vi "SynthNV_2_5c.vi"() -> ()   [LabVIEW 2012]
uses:
  <vilib>/Utility/error.llb/DialogType.ctl
  <vilib>/Instr/_visa.llb/VISA Flush IO Buffer Mask.ctl
  <vilib>/Utility/file.llb/Read From Spreadsheet File (DBL).vi
  <vilib>/Instr/_visa.llb/VISA Configure Serial Port (Instr).vi
panel:
  out "Power (dBm)":dbl format="%#_4g"
  out "caldata":dbl[][](array[numeric]) format="%0.3f"
  out "COM Error":bool
  out "Device Under Control":string
  in  "Boolean":bool
  in  "Serial Port Select":refnum<visa-resource-name>="COM3"
  in  "Load":bool
  out "Lock":bool
  in  "RF HP":bool=TRUE
  in  "RF On":bool=TRUE
  in  "Dial Tab":enum32{"VFO Dial", "Touch Pad"}(tab)
  in  "Frequency Adjust":i8(knob)=1 scale=1.0..20.0
  in  "Knob Step Size":i32(ring)=3 items=["1KHz", "10KHz", "100KHz", "1MHz", "10MHz", "100MHz", "1GHz"]
  out "Freq (MHz) 3":dbl format="%#_7g"
  in  "KeyPad":T1
  out "KeyPad Out":dbl format="%7_7g"
  in  "Attenuator (dB)":dbl(slide)=-31.5 min=-31.5 max=0.0 step=0.5
  in  "stop":bool
  in  "Tab Control":T2(tab)
  in  "RF  FREQUENCY MHz":dbl=1000.0 min=34.375 max=4400.0 step=1.0 format="%_7g"
  in  "Enter":bool caption="1"
  out "PWR Level":bool
  out "Waveform Chart":dbl(graph)
  out "RF Detector Pwr dBm":dbl=-67.9609375 format="%_5g"
  in  "Read Power":bool
  in  "VREF":dbl=2.52 format="%#_7g"
  in  "POFFSET":dbl=97.0 format="%#_7g"
  in  "Send\nCal":bool
  in  "Start Network\nAnalyzer":bool
  out "Number\nof Points":dbl format="%#.6g"
  in  "Stop Frequency":dbl=4000.0 min=34.0 max=4400.0 step=0.001 format="%7_7g"
  in  "Step Time (mS)":dbl=0.55 min=0.25 max=10000.0 step=1.0 format="%_8g"
  in  "Step Size MHz":dbl=50.0 min=0.001 max=4200.0 step=1.0 format="%#_7f"
  in  "Enter SZ":bool caption="1"
  in  "Enter Start":bool caption="1"
  in  "Enter Stop":bool caption="1"
  in  "Enter ST":bool caption="1"
  in  "Start Frequency":dbl=50.0 min=34.0 max=4400.0 step=0.001 format="%7_7g"
  in  "Sweep\nOnce":bool
  in  "Sweep\nContinuously":bool
  in  "Mod Tab":enum32{"PULSE Amplitude", "AM"}(tab)
  in  "Mod Style":bool
  in  "PULNUM":bool caption="1"
  in  "PULOFF":bool caption="1"
  in  "PULON":bool caption="1"
  in  "Send Pulse Burst":bool
  out "Duration (uS)":dbl
  in  "Continuous PM":bool
  in  "# of Pulses":u16=100 min=1 step=1 format="%#.5f"
  in  "Off Time (uS)":u16=10 min=1 max=16000 step=1 format="%#.5f"
  in  "On Time (uS)":u16=1 min=1 max=16000 step=1 format="%#.5f"
  in  "AMAMP":bool caption="1"
  in  "AMPWR":bool caption="1"
  in  "AMCYC":bool caption="1"
  in  "AMFREQ":bool caption="1"
  in  "AM Freq (Hz)":dbl=1000.0 min=2.0 max=500000.0 step=10.0 format="%#.6f"
  out "Actual Freq (Hz)":dbl
  out "Duration (ms)":dbl
  in  "Send AM Burst":bool
  in  "# of Cycles":u16=100 min=1 step=1 format="%#.5f"
  in  "Offset":u8 max=62 step=1
  in  "Amplitude (%)":u8=100 min=1 max=100 step=1
  in  "Continuous AM":bool
  in  "Wave Shape":u8(ring) items=["Sine", "Ramp", "Triangle"]
  in  "LUTsize":u8=32 min=2 step=1
  in  "Read Settings\nFrom SynthNV":bool
  out "read buffer":string
  in  "Allow changing\nof Power Detector\ncalibration values":bool
  in  "GP Dig Out J8 P3":bool
  in  "Read A/D \non J8 P2":bool
  in  "Read A/D \non J8 P1":bool
  in  "REF":bool=TRUE
  in  "Program\nEEprom":bool
  in  "Read\nFirmware\nVersion":bool
  out "Version":string
  in  "Program\nReference":bool
  in  "Poll for\nPhase Lock":bool
  out "A/D1":string
  out "A/D2":string
  in  "GP Dig Out J8 P5":bool
  out "Frac":i32
  out "Modulus":i32=500
  out "INT":i16=2000
  out "RF Divider":i32=4
  out "Allregout":u32[](array[numeric])=[4194309, 10896444, 1203, 97986, 134254497, 65536000] format="%08x"
  out "PFd(MHz)":dbl=2.0
  in  "PllCntrl":T3={"PLL PWR"=3, "MUX out"=4, "Phase"=1, "Low Noise"=TRUE, "REF X2"=FALSE, "Mute till LD"=TRUE, "Icp"=15, "Band Sel Div"=16, "REF Divide"=5, "Reference(MHz)"=10.0} {"Icp" scale=0.0..15.0; "MUX out" items=["3-State", "GND", "Vcc", "Analog LD", "Digital LD", "REF / R", "RF / N"]; "PLL PWR" scale=0.0..3.0}
  in  "Step Size (MHz)":dbl=0.001
  in  "Send":bool
  in  "Freq (MHz)":dbl=1000.0 format="%_10g"
  in  "Re-init\nDefaults":bool
  # "v2.5c"
  # "Windfreak Technologies"
  # "MHz"
  # "Windfreak Technologies, LLC 2012"
  # "Warning: Max RF power into the\ndetector is 10dBm.  The Synthesizer\ncan generate up to +20dBm.  \nPlease use an external attenuator."
  # "Burst"
  # "Peak Amplitude is\nadjusted with slider\nbar on the right"
  # "Adjust Power Slider to get CW\npower back on after a pulse."
  # "Burst"
  # "(Or Update)"
  # "(Watch for LED D3 toggle.)"
  # "This Tab is for experimental purposes only."
  # "RF Freq (MHz)"
  # "REG5"
  # "REG4"
  # "REG3"
  # "REG2"
  # "REG1"
  # "REG0"
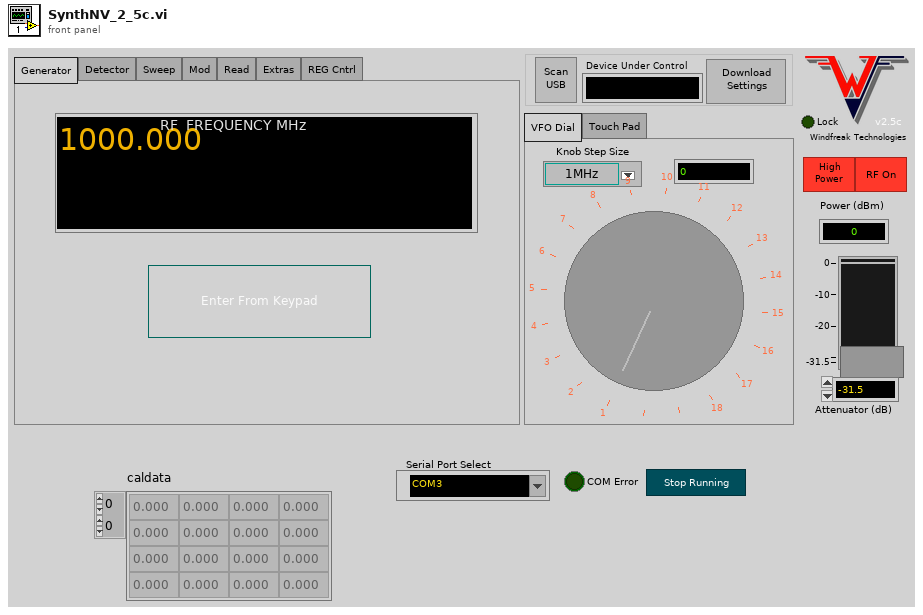
[diagram p1: front panel]
types:
  T1 = cluster{"2":bool, "1":bool, "3":bool, "4":bool, "9":bool, "5":bool, "6":bool, "7":bool, "8":bool, "0":bool, "dp":bool, "Clear":bool}
  T2 = enum32{"Generator", "Detector", "Sweep", "Mod", "Read", "Extras", "REG Cntrl"}
  T3 = cluster{"PLL PWR":i8, "MUX out":u16, "Phase":i16, "Low Noise":bool, "REF X2":bool, "Mute till LD":bool, "Icp":i32, "Band Sel Div":i32, "REF Divide":i16, "Reference(MHz)":dbl}
  T4 = enum8{"Enabled", "Disabled", "Disabled and Grayed Out"}
  T5 = typedef "DialogType.ctl" = u16
  T6 = typedef "VISA Flush IO Buffer Mask.ctl" = u16
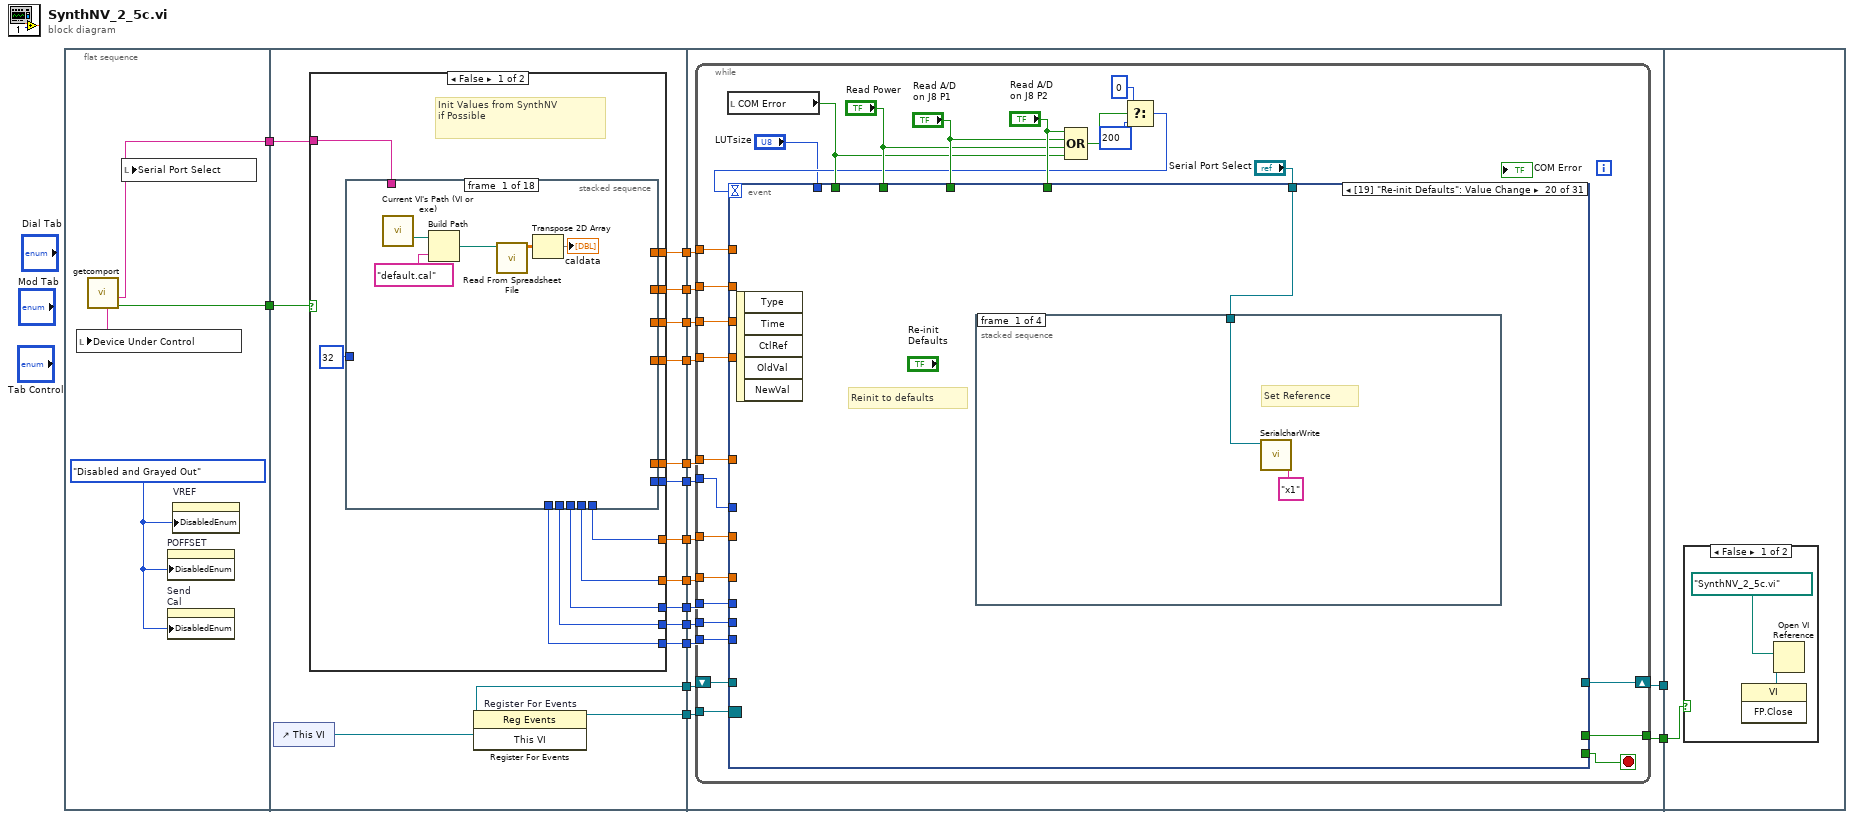
[diagram p0: block diagram]
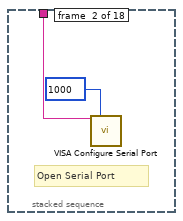
[diagram p2: hidden frame]
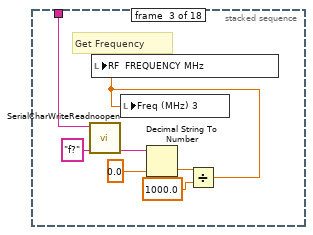
[diagram p3: hidden frame]
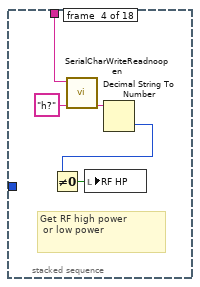
[diagram p4: hidden frame]
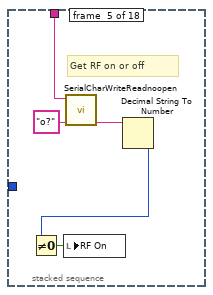
[diagram p5: hidden frame]
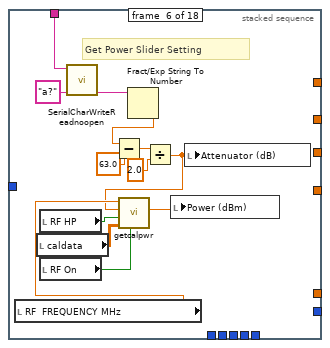
[diagram p6: hidden frame]
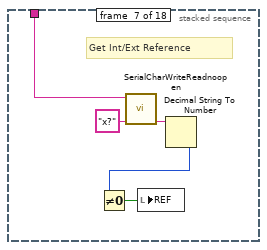
[diagram p7: hidden frame]
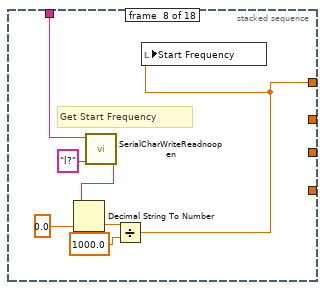
[diagram p8: hidden frame]
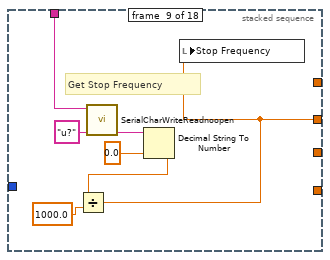
[diagram p9: hidden frame]
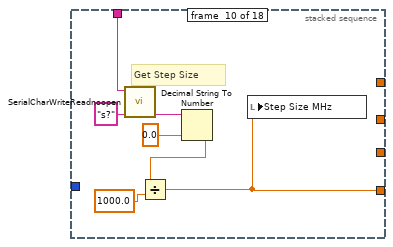
[diagram p10: hidden frame]
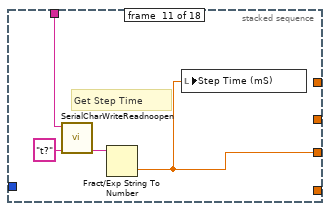
[diagram p11: hidden frame]
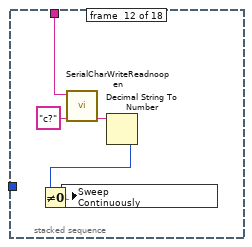
[diagram p12: hidden frame]
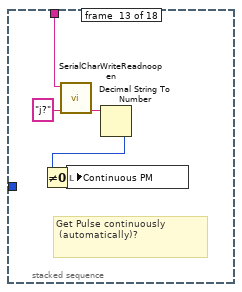
[diagram p13: hidden frame]
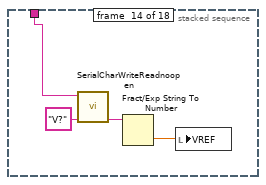
[diagram p14: hidden frame]
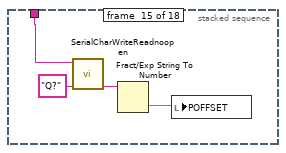
[diagram p15: hidden frame]
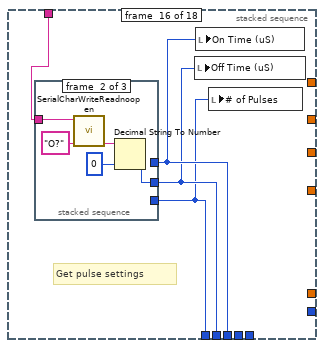
[diagram p16: hidden frame]
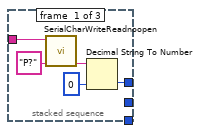
[diagram p17: hidden frame]
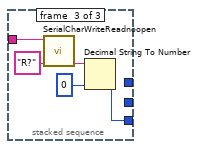
[diagram p18: hidden frame]
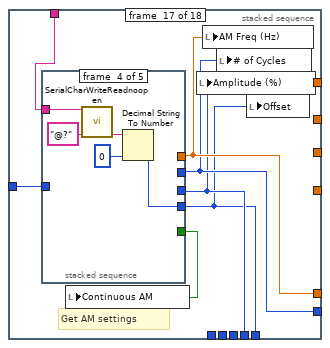
[diagram p19: hidden frame]
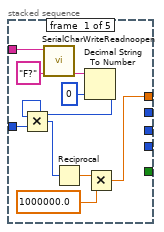
[diagram p20: hidden frame]
diagram:
  n1 = flat-sequence {
    tunnel: [w21] -> w17
    tunnel: [w20] -> w5
    tunnel: w17 -> [w36]
    tunnel: [w35] -> w16
    tunnel: [w34] -> w15
    tunnel: [w33] -> w14
    tunnel: [w32] -> w13
    tunnel: [w31] -> w12
    tunnel: [w30] -> w11
    tunnel: [w29] -> w10
    tunnel: [w28] -> w9
    tunnel: [w27] -> w8
    tunnel: [w26] -> w7
    tunnel: [w25] -> w6
    tunnel: w5 -> [w24]
    tunnel: [w22] -> w4
    tunnel: [w23] -> w3
    tunnel: w16 -> [w224]
    tunnel: w15 -> [w223]
    tunnel: w14 -> [w222]
    tunnel: w13 -> [w221]
    tunnel: w12 -> [w220]
    tunnel: w11 -> [w219]
    tunnel: w10 -> [w218]
    tunnel: w9 -> [w217]
    tunnel: w8 -> [w216]
    tunnel: w7 -> [w215]
    tunnel: w6 -> [w214]
    tunnel: w4 -> [w212]
    tunnel: w3 -> [w213]
    tunnel: [w211] -> w2
    tunnel: [w210] -> w1
    tunnel: w2 -> [_]
    tunnel: w1 -> [w887]
    frame #0 {
      w18 = T4."Disabled and Grayed Out" ("Disabled")
      n2 = call "getcomport.vi"() -> ("No Devices"=w21:bool, "Port"=w20:string, "Device"=w19:string)  [unwired: 9 in]
      n3 = local write "Device Under Control"(w19) -> ()
      n4 = local write "Serial Port Select"(w20) -> ()
      n5 = property on="POFFSET" class="DigNum (strict)"("DisabledEnum"=w18) -> ()  [unwired: 2 in, 2 out]
      n6 = property on="Send\nCal" class="Bool"("DisabledEnum"=w18) -> ()  [unwired: 2 in, 2 out]
      n7 = property on="VREF" class="DigNum (strict)"("DisabledEnum"=w18) -> ()  [unwired: 2 in, 2 out]
    }
    frame #1 {
      n8 = control-ref of="This VI"() -> (w23:refnum<vi>)
      n9 = case shown="False" w36 {
        tunnel: [w48 200.0 ("Start ini")] -> w35
        tunnel: [w47 4000.0 ("upper limit")] -> w34
        tunnel: [w45 u32 5 ("upper limit")] -> w33
        tunnel: [w46 50.0 ("upper limit")] -> w32
        tunnel: [w37 1000.0 ("Amp ini")] -> w31
        tunnel: [w38 u16 100 ("OnT ini")] -> w30
        tunnel: [w40 0.0 ("Amp ini")] -> w29
        tunnel: [w39 31.5 ("Amp ini")] -> w28
        tunnel: [w44 u16 1 ("OnT ini")] -> w27
        tunnel: [w42 u16 15 ("OnT ini")] -> w26
        tunnel: [w43 u16 100 ("OnT ini")] -> w25
        tunnel: w24 -> [w49 _]
        frame False {
          # "Init Values from SynthNV\nif Possible"
          n10 = stacked-sequence {
            tunnel: w49 -> [_ w56 w63 w65 w71 w84 w88 w93 w100 w107 w115 w118 w123 w128 w132 w138 w160 w192]
            tunnel: u8 32 ("LUTsize") -> [_ _ _ _ _ _ _ _ _ _ _ _ _ _ _ _ w159 _]
            tunnel: [_ _ _ _ _ _ _ w92 _ _ _ _ _ _ _ _ _ _] -> w48
            tunnel: [_ _ _ _ _ _ _ _ w99 _ _ _ _ _ _ _ _ _] -> w47
            tunnel: [_ _ _ _ _ _ _ _ _ w106 _ _ _ _ _ _ _ _] -> w46
            tunnel: [_ _ _ _ _ _ _ _ _ _ w113 _ _ _ _ _ _ _] -> w45
            tunnel: [_ _ _ _ _ _ _ _ _ _ _ _ _ _ _ w137 _ _] -> w44
            tunnel: [_ _ _ _ _ _ _ _ _ _ _ _ _ _ _ w135 _ _] -> w43
            tunnel: [_ _ _ _ _ _ _ _ _ _ _ _ _ _ _ w136 _ _] -> w42
            tunnel: [_ _ _ _ _ _ _ _ _ _ _ _ _ _ _ _ w154 _] -> w40
            tunnel: [_ _ _ _ _ _ _ _ _ _ _ _ _ _ _ _ w155 _] -> w39
            tunnel: [_ _ _ _ _ _ _ _ _ _ _ _ _ _ _ _ w156 _] -> w38
            tunnel: [_ _ _ _ _ _ _ _ _ _ _ _ _ _ _ _ w157 _] -> w37
            frame #0 {
              n11 = call "Current VI's Path (VI or exe).vi"() -> ("VI or executable installation directory"=w50:path)  [unwired: 14 in, 1 out]
              n12 = Build Path(base path=w50, name or relative path="default.cal") -> (appended path=w53:path)
              n13 = call-poly <vilib>:"Read From Spreadsheet File.vi"("file path (dialog if empty)"=w53) -> ("all rows"=w51:dbl[][])  [unwired: 6 in, 4 out]
              n14 = Transpose 2D Array(2D array=w51) -> (transposed array=→"caldata":dbl[][])
            }
            frame #1 {
              # "Open Serial Port"
              n15 = call-poly "VISA Configure Serial Port"("VISA resource name"=w56, "timeout (10sec)"=u32 1000) -> ()  [unwired: 7 in, 7 out]
            }
            frame #2 {
              # "Get Frequency"
              n16 = call "SerialCharWriteReadnoopen.vi"("VISA resource name"=w63, "write buffer"="f?") -> ("read buffer"=w61:string)  [unwired: 8 in]
              n17 = Decimal String To Number(string=w61, default (0L)=0.0 ("default (0 I32)")) -> (number=w59:dbl)  [unwired: 1 in, 1 out]
              n18 = Divide(x=w59, y=1000.0) -> (x/y=w57:dbl)
              n19 = local write "RF  FREQUENCY MHz"(w57) -> ()
              n20 = local write "Freq (MHz) 3"(w57) -> ()
            }
            frame #3 {
              # "Get RF high power\n or low power"
              n21 = call "SerialCharWriteReadnoopen.vi"("VISA resource name"=w65, "write buffer"="h?") -> ("read buffer"=w67:string)  [unwired: 8 in]
              n22 = Decimal String To Number(string=w67) -> (number=w66:i32)  [unwired: 2 in, 1 out]
              n23 = Not Equal To 0?(x=w66) -> (x != 0?=w64:bool)
              n24 = local write "RF HP"(w64) -> ()
            }
            frame #4 {
              # "Get RF on or off"
              n25 = call "SerialCharWriteReadnoopen.vi"("VISA resource name"=w71, "write buffer"="o?") -> ("read buffer"=w72:string)  [unwired: 8 in]
              n26 = Decimal String To Number(string=w72) -> (number=w70:i32)  [unwired: 2 in, 1 out]
              n27 = Not Equal To 0?(x=w70) -> (x != 0?=w69:bool)
              n28 = local write "RF On"(w69) -> ()
            }
            frame #5 {
              # "Get Power Slider Setting"
              n29 = local read "RF  FREQUENCY MHz"() -> (w78:dbl)
              n30 = local read "caldata"() -> (w79:dbl[][])
              n31 = local read "RF HP"() -> (w76:bool)
              n32 = local read "RF On"() -> (w75:bool)
              n33 = call "SerialCharWriteReadnoopen.vi"("VISA resource name"=w84, "write buffer"="a?") -> ("read buffer"=w85:string)  [unwired: 8 in]
              n34 = Fract/Exp String To Number(string=w85) -> (number=w80:dbl)  [unwired: 3 in, 1 out]
              n35 = Subtract(x=w80, y=63.0) -> (x-y=w81:dbl)
              n36 = Divide(x=w81, y=2.0) -> (x/y=w74:dbl)
              n37 = call "getcalpwr.vi"("RF On"=w75, "caldata"=w79, "RF HP"=w76, "attn"=w74, "freq"=w78) -> ("actual"=w77:dbl)  [unwired: 5 in]
              n38 = local write "Power (dBm)"(w77) -> ()
              n39 = local write "Attenuator (dB)"(w74) -> ()
            }
            frame #6 {
              # "Get Int/Ext Reference"
              n40 = call "SerialCharWriteReadnoopen.vi"("VISA resource name"=w88, "write buffer"="x?") -> ("read buffer"=w90:string)  [unwired: 8 in]
              n41 = Decimal String To Number(string=w90) -> (number=w89:i32)  [unwired: 2 in, 1 out]
              n42 = Not Equal To 0?(x=w89) -> (x != 0?=w87:bool)
              n43 = local write "REF"(w87) -> ()
            }
            frame #7 {
              # "Get Start Frequency"
              n44 = call "SerialCharWriteReadnoopen.vi"("VISA resource name"=w93, "write buffer"="l?") -> ("read buffer"=w97:string)  [unwired: 8 in]
              n45 = Decimal String To Number(string=w97, default (0L)=0.0 ("default (0 I32)")) -> (number=w95:dbl)  [unwired: 1 in, 1 out]
              n46 = Divide(x=w95, y=1000.0) -> (x/y=w92:dbl)
              n47 = local write "Start Frequency"(w92) -> ()
            }
            frame #8 {
              # "Get Stop Frequency"
              n48 = call "SerialCharWriteReadnoopen.vi"("VISA resource name"=w100, "write buffer"="u?") -> ("read buffer"=w104:string)  [unwired: 8 in]
              n49 = Decimal String To Number(string=w104, default (0L)=0.0 ("default (0 I32)")) -> (number=w102:dbl)  [unwired: 1 in, 1 out]
              n50 = Divide(x=w102, y=1000.0) -> (x/y=w99:dbl)
              n51 = local write "Stop Frequency"(w99) -> ()
            }
            frame #9 {
              # "Get Step Size"
              n52 = call "SerialCharWriteReadnoopen.vi"("VISA resource name"=w107, "write buffer"="s?") -> ("read buffer"=w111:string)  [unwired: 8 in]
              n53 = Decimal String To Number(string=w111, default (0L)=0.0 ("default (0 I32)")) -> (number=w109:dbl)  [unwired: 1 in, 1 out]
              n54 = Divide(x=w109, y=1000.0) -> (x/y=w106:dbl)
              n55 = local write "Step Size MHz"(w106) -> ()
            }
            frame #10 {
              # "Get Step Time"
              n56 = call "SerialCharWriteReadnoopen.vi"("VISA resource name"=w115, "write buffer"="t?") -> ("read buffer"=w114:string)  [unwired: 8 in]
              n57 = Fract/Exp String To Number(string=w114) -> (number=w113:dbl)  [unwired: 3 in, 1 out]
              n58 = local write "Step Time (mS)"(w113) -> ()
            }
            frame #11 {
              n59 = call "SerialCharWriteReadnoopen.vi"("VISA resource name"=w118, "write buffer"="c?") -> ("read buffer"=w120:string)  [unwired: 8 in]
              n60 = Decimal String To Number(string=w120) -> (number=w119:i32)  [unwired: 2 in, 1 out]
              n61 = Not Equal To 0?(x=w119) -> (x != 0?=w117:bool)
              n62 = local write "Sweep\nContinuously"(w117) -> ()
            }
            frame #12 {
              # "Get Pulse continuously\n (automatically)?"
              n63 = call "SerialCharWriteReadnoopen.vi"("VISA resource name"=w123, "write buffer"="j?") -> ("read buffer"=w125:string)  [unwired: 8 in]
              n64 = Decimal String To Number(string=w125) -> (number=w124:i32)  [unwired: 2 in, 1 out]
              n65 = Not Equal To 0?(x=w124) -> (x != 0?=w122:bool)
              n66 = local write "Continuous PM"(w122) -> ()
            }
            frame #13 {
              n67 = call "SerialCharWriteReadnoopen.vi"("VISA resource name"=w128, "write buffer"="V?") -> ("read buffer"=w129:string)  [unwired: 8 in]
              n68 = Fract/Exp String To Number(string=w129) -> (number=w127:dbl)  [unwired: 3 in, 1 out]
              n69 = local write "VREF"(w127) -> ()
            }
            frame #14 {
              n70 = call "SerialCharWriteReadnoopen.vi"("VISA resource name"=w132, "write buffer"="Q?") -> ("read buffer"=w133:string)  [unwired: 8 in]
              n71 = Fract/Exp String To Number(string=w133) -> (number=w131:dbl)  [unwired: 3 in, 1 out]
              n72 = local write "POFFSET"(w131) -> ()
            }
            frame #15 {
              # "Get pulse settings"
              n73 = stacked-sequence {
                tunnel: w138 -> [w141 w146 w151]
                tunnel: [w139 _ _] -> w137
                tunnel: [_ w145 _] -> w136
                tunnel: [_ _ w150] -> w135
                frame #0 {
                  n74 = call "SerialCharWriteReadnoopen.vi"("VISA resource name"=w141, "write buffer"="P?") -> ("read buffer"=w142:string)  [unwired: 8 in]
                  n75 = Decimal String To Number(string=w142, default (0L)=u16 0 ("default (0 I32)")) -> (number=w139:u16)  [unwired: 1 in, 1 out]
                }
                frame #1 {
                  n76 = call "SerialCharWriteReadnoopen.vi"("VISA resource name"=w146, "write buffer"="O?") -> ("read buffer"=w147:string)  [unwired: 8 in]
                  n77 = Decimal String To Number(string=w147, default (0L)=u16 0 ("default (0 I32)")) -> (number=w145:u16)  [unwired: 1 in, 1 out]
                }
                frame #2 {
                  n78 = call "SerialCharWriteReadnoopen.vi"("VISA resource name"=w151, "write buffer"="R?") -> ("read buffer"=w152:string)  [unwired: 8 in]
                  n79 = Decimal String To Number(string=w152, default (0L)=u16 0 ("default (0 I32)")) -> (number=w150:u16)  [unwired: 1 in, 1 out]
                }
              }
              n80 = local write "Off Time (uS)"(w136) -> ()
              n81 = local write "On Time (uS)"(w137) -> ()
              n82 = local write "# of Pulses"(w135) -> ()
            }
            frame #16 {
              # "Get AM settings"
              n83 = stacked-sequence {
                tunnel: w160 -> [w168 w173 w178 w182 w186]
                tunnel: [_ w172 _ _ _] -> w156
                tunnel: [_ _ w177 _ _] -> w155
                tunnel: [_ _ _ w181 _] -> w154
                tunnel: w159 -> [w166 _ _ _ _]
                tunnel: [w161 _ _ _ _] -> w157
                tunnel: [_ _ _ _ w187] -> w158
                frame #0 {
                  n84 = call "SerialCharWriteReadnoopen.vi"("VISA resource name"=w168, "write buffer"="F?") -> ("read buffer"=w169:string)  [unwired: 8 in]
                  n85 = Decimal String To Number(string=w169, default (0L)=u16 0 ("default (0 I32)")) -> (number=w165:u16)  [unwired: 1 in, 1 out]
                  n86 = Multiply(x=w165, y=w166) -> (x*y=w164:u16)
                  n87 = Reciprocal(x=w164) -> (1/x=w163:dbl)
                  n88 = Multiply(x=w163, y=1000000.0) -> (x*y=w161:dbl)
                }
                frame #1 {
                  n89 = call "SerialCharWriteReadnoopen.vi"("VISA resource name"=w173, "write buffer"="q?") -> ("read buffer"=w174:string)  [unwired: 8 in]
                  n90 = Decimal String To Number(string=w174, default (0L)=u16 0 ("default (0 I32)")) -> (number=w172:u16)  [unwired: 1 in, 1 out]
                }
                frame #2 {
                  n91 = call "SerialCharWriteReadnoopen.vi"("VISA resource name"=w178, "write buffer"="%?") -> ("read buffer"=w179:string)  [unwired: 8 in]
                  n92 = Decimal String To Number(string=w179, default (0L)=u16 0 ("default (0 I32)")) -> (number=w177:u16)  [unwired: 1 in, 1 out]
                }
                frame #3 {
                  n93 = call "SerialCharWriteReadnoopen.vi"("VISA resource name"=w182, "write buffer"="@?") -> ("read buffer"=w184:string)  [unwired: 8 in]
                  n94 = Decimal String To Number(string=w184, default (0L)=u16 0 ("default (0 I32)")) -> (number=w181:u16)  [unwired: 1 in, 1 out]
                }
                frame #4 {
                  # "Cont AM"
                  n95 = call "SerialCharWriteReadnoopen.vi"("VISA resource name"=w186, "write buffer"="A?") -> ("read buffer"=w189:string)  [unwired: 8 in]
                  n96 = Decimal String To Number(string=w189) -> (number=w190:i32)  [unwired: 2 in, 1 out]
                  n97 = Not Equal To 0?(x=w190) -> (x != 0?=w187:bool)
                }
              }
              n98 = local write "Continuous AM"(w158) -> ()
              n99 = local write "Amplitude (%)"(w155) -> ()
              n100 = local write "AM Freq (Hz)"(w157) -> ()
              n101 = local write "# of Cycles"(w156) -> ()
              n102 = local write "Offset"(w154) -> ()
            }
            frame #17 {
              w196 = T5 0 items=["no dialog", "OK message", "continue or stop message", "OK message + warnings", "continue/stop + warnings"] ("type of dialog (OK msg:1)")
              # "Close session to port."
              n103 = VISA Close(VISA resource name=w192) -> (error out=w197:errorcluster)  [unwired: 1 in]
              n104 = call <vilib>:"Simple Error Handler.vi"("type of dialog (OK msg:1)"=w196, "error in (no error)"=w197) -> ("error?"=w191:bool)  [unwired: 7 out]
              n105 = Equal?(x=w191, y=TRUE) -> (x = y?=w194:bool)
              n106 = case shown="True" w194 {
                tunnel: "Serial Port Error" ("message") -> [_ w198]
                frame False {
                }
                frame True {
                  n107 = Two Button Dialog(message=w198) -> ()  [unwired: 2 in, 1 out]
                }
              }
            }
          }
        }
        frame True {
        }
      }
      n108 = register-events "Register For Events"(w23) -> (reference out=w22:refnum<event-registration>)  [unwired: 2 in, 1 out]
    }
    frame #2 {
      n109 = while {
        tunnel: w223 -> [w250]
        tunnel: w222 -> [w249]
        tunnel: w221 -> [w248]
        tunnel: w224 -> [w247]
        tunnel: w220 -> [w246]
        tunnel: w219 -> [w245]
        tunnel: w218 -> [w240]
        tunnel: w217 -> [w244]
        tunnel: w216 -> [w243]
        tunnel: w215 -> [w242]
        tunnel: w214 -> [w241]
        shift-right: [w235] -> w211
        shift-left: w213 -> [w237]
        tunnel: w212 -> [w236]
        tunnel: [w234] -> w210
        stop <- w238 stop-if-true
        n110 = local read "COM Error"() -> (w228:bool)
        n111 = Compound Arithmetic op=OR("Read A/D \non J8 P2", "Read A/D \non J8 P1", "Read Power", w228) -> (w227:bool)
        n112 = Select(t=0, s=w227, f=200) -> (s? t:f=w226:i32)
        n113 = event shown="[19] \"Re-init Defaults\": Value Change" {
          selector: w236 -> [_ _ _ _ _ _ _ _ _ _ _ _ _ _ _ _ _ _ _ _ _ _ _ _ _ _ _ _ _ _ _]
          dyn-events: _ -> [_ _ _ _ _ _ _ _ _ _ _ _ _ _ _ _ _ _ _ _ _ _ _ _ _ _ _ _ _ _ _]
          timeout: w226 -> [_ _ _ _ _ _ _ _ _ _ _ _ _ _ _ _ _ _ _ _ _ _ _ _ _ _ _ _ _ _ _]
          tunnel: w250 -> [_ w300 _ _ _ _ _ _ _ _ _ _ _ _ _ _ _ _ _ _ _ _ _ _ _ _ _ _ _ _ _]
          tunnel: w249 -> [_ w299 _ _ _ _ _ _ _ _ _ _ _ _ _ _ _ _ _ _ _ _ _ _ _ _ _ _ _ _ _]
          tunnel: w248 -> [_ w298 _ _ _ _ _ _ _ _ _ _ _ _ _ _ _ _ _ _ _ _ _ _ _ _ _ _ _ _ _]
          tunnel: w247 -> [_ w297 _ _ _ _ _ _ _ _ _ _ _ _ _ _ _ _ _ _ _ _ _ _ _ _ _ _ _ _ _]
          tunnel: w246 -> [_ w276 _ _ _ _ _ _ _ _ _ _ _ _ _ _ _ _ _ _ _ _ _ _ _ _ _ _ _ _ _]
          tunnel: w245 -> [_ w275 _ _ _ _ _ _ _ _ _ _ _ _ _ _ _ _ _ _ _ _ _ _ _ _ _ _ _ _ _]
          tunnel: w244 -> [_ w274 _ _ _ _ _ _ _ _ _ _ _ _ _ _ _ _ _ _ _ _ _ _ _ _ _ _ _ _ _]
          tunnel: w243 -> [_ w267 _ _ _ _ _ _ _ _ _ _ _ _ _ _ _ _ _ _ _ _ _ _ _ _ _ _ _ _ _]
          tunnel: w242 -> [_ w268 _ _ _ _ _ _ _ _ _ _ _ _ _ _ _ _ _ _ _ _ _ _ _ _ _ _ _ _ _]
          tunnel: w241 -> [_ w273 _ _ _ _ _ _ _ _ _ _ _ _ _ _ _ _ _ _ _ _ _ _ _ _ _ _ _ _ _]
          tunnel: w240 -> [_ w270 _ _ _ _ _ _ _ _ _ _ _ _ _ _ _ _ _ _ _ _ _ _ _ _ _ _ _ _ _]
          tunnel: "Serial Port Select" -> [w263 _ w312 w327 w354 w401 w402 _ w415 w426 _ w437 w441 w449 w456 w462 w465 w474 w489 w565 w594 w595 w602 w605 w616 w625 w638 w650 _ _ w841]
          tunnel: [_ _ _ _ _ _ _ "stop" _ _ _ _ _ _ _ _ _ _ _ _ _ _ _ _ _ _ _ _ _ w835 _] -> w238
          tunnel: w237 -> [_ _ _ _ _ _ _ _ _ _ _ _ _ _ _ _ _ _ _ _ _ _ _ _ _ _ _ _ _ w834 _]
          tunnel: [_ _ _ _ _ _ _ _ _ _ _ _ _ _ _ _ _ _ _ _ _ _ _ _ _ _ _ _ _ w834 _] -> w235
          tunnel: [_ _ _ _ _ _ _ "stop" _ _ _ _ _ _ _ _ _ _ _ _ _ _ _ _ _ _ _ _ _ _ _] -> w234
          tunnel: w228 -> [_ _ _ _ _ _ _ _ _ _ _ _ _ _ _ _ _ _ _ _ _ _ _ _ _ _ _ _ _ _ w840]
          tunnel: "Read Power" -> [_ _ _ _ _ _ _ _ _ _ _ _ _ _ _ _ _ _ _ _ _ _ _ _ _ _ _ _ _ _ w839]
          tunnel: "Read A/D \non J8 P1" -> [_ _ _ _ _ _ _ _ _ _ _ _ _ _ _ _ _ _ _ _ _ _ _ _ _ _ _ _ _ _ w838]
          tunnel: "Read A/D \non J8 P2" -> [_ _ _ _ _ _ _ _ _ _ _ _ _ _ _ _ _ _ _ _ _ _ _ _ _ _ _ _ _ _ w837]
          tunnel: "LUTsize" -> [_ _ _ _ _ _ _ _ _ _ _ _ _ _ _ w457 w464 _ _ _ _ _ _ _ _ _ _ _ w670 _ _]
          event "Frequency Adjust", "RF  FREQUENCY MHz": Value Change {
            n114 = event-data() -> ()  [unwired: 1 in, 5 out]
            n115 = call "Knob.vi"("Freqin"="RF  FREQUENCY MHz", "Knob"="Frequency Adjust", "Knob Step Size"="Knob Step Size") -> ("Freqout"=w256:dbl)  [unwired: 7 in]
            "Freq (MHz) 3" <- w256
            n116 = local write "RF  FREQUENCY MHz"(w256) -> ()
            n117 = local read "Attenuator (dB)"() -> (w251:dbl)
            n118 = local read "caldata"() -> (w255:dbl[][])
            n119 = local read "RF HP"() -> (w253:bool)
            n120 = local read "RF On"() -> (w252:bool)
            n121 = Number To Fractional String(use system decimal point (T)=FALSE, number=w256, precision (6)=i16 3) -> (F-format string=w261:string)  [unwired: 1 in]
            n122 = call "getcalpwr.vi"("RF On"=w252, "caldata"=w255, "RF HP"=w253, "attn"=w251, "freq"=w256) -> ("actual"=w254:dbl)  [unwired: 5 in]
            n123 = Concatenate Strings("f" ("element"), w261) -> (w258:string)
            n124 = local write "Power (dBm)"(w254) -> ()
            n125 = call "SerialcharWrite.vi"("VISA resource name"=w263, "write buffer"=w258) -> ("ComError"=w262:bool)  [unwired: 8 in]
            n126 = local write "COM Error"(w262) -> ()
          }
          event "AMPWR", "AMCYC", "Enter Start", "Enter Stop", "Enter ST", "Enter SZ", "AMAMP", "AMFREQ", "PULNUM", "PULOFF", "PULON": Value Change {
            n127 = event-data() -> ()  [unwired: 1 in, 5 out]
            n128 = local read "KeyPad Out"() -> (w269:dbl)
            n129 = call "PulseModEntry.vi"("OnTimeSet"="PULON", "Keypad In"=w269, "OnT ini"=w267, "OffTimeSet"="PULOFF", "OffT ini"=w268, "PulsesSet"="PULNUM", "Pulses ini"=w273) -> ("OnTime"=w284:u16, "OffTime"=w283:u16, "NumPulses"=w271:u32)  [unwired: 4 in, 2 out]
            n130 = call "AMModEntry.vi"("AMFreqSet"="AMFREQ", "Keypad In"=w269, "AMFreq ini"=w276, "NumCycSet"="AMCYC", "NumCyc ini"=w275, "PkPwrSet"="AMPWR", "PkPwr ini"=w270, "AmpSet"="AMAMP", "Amp ini"=w274) -> ("AM Freq"=w288:dbl, "NumCyc"=w287:u16, "PkPwr"=w286:dbl, "Amplitude"=w285:dbl)  [unwired: 2 in, 1 out]
            n131 = call "SweepDataEntry.vi"("Enter Stop"="Enter Stop", "Start ini"=w297, "Enter Start"="Enter Start", "Keypad In"=w269, "Stop ini"=w300, "Enter ST"="Enter ST", "Step ini"=w299, "Enter SZ"="Enter SZ", "SZ ini"=w298) -> ("START FREQUENCY MHz"=w291:dbl, "STOP FREQUENCY MHz"=w292:dbl, "Step Time mS"=w293:dbl, "Step Size MHz"=w294:dbl)  [unwired: 2 in, 1 out]
            n132 = case shown="True" "Enter ST" {
              tunnel: w293 -> [_ w309]
              frame False {
              }
              frame True {
                n133 = local write "Step Time (mS)"(w309) -> ()
              }
            }
            n134 = case shown="True" "Enter SZ" {
              tunnel: w294 -> [_ w308]
              frame False {
              }
              frame True {
                n135 = local write "Step Size MHz"(w308) -> ()
              }
            }
            n136 = case shown="True" "Enter Start" {
              tunnel: w291 -> [_ w311]
              frame False {
              }
              frame True {
                n137 = local write "Start Frequency"(w311) -> ()
              }
            }
            n138 = case shown="True" "Enter Stop" {
              tunnel: w292 -> [_ w310]
              frame False {
              }
              frame True {
                n139 = local write "Stop Frequency"(w310) -> ()
              }
            }
            n140 = case shown="True" "AMAMP" {
              tunnel: w285 -> [_ w304]
              frame False {
              }
              frame True {
                n141 = local write "Amplitude (%)"(w304) -> ()
              }
            }
            n142 = case shown="True" "AMFREQ" {
              tunnel: w288 -> [_ w307]
              frame False {
              }
              frame True {
                n143 = local write "AM Freq (Hz)"(w307) -> ()
              }
            }
            n144 = case shown="True" "AMCYC" {
              tunnel: w287 -> [_ w306]
              frame False {
              }
              frame True {
                n145 = local write "# of Cycles"(w306) -> ()
              }
            }
            n146 = case shown="True" "AMPWR" {
              tunnel: w286 -> [_ w305]
              frame False {
              }
              frame True {
                n147 = local write "Offset"(w305) -> ()
              }
            }
            n148 = case shown="True" "PULON" {
              tunnel: w284 -> [_ w303]
              frame False {
              }
              frame True {
                n149 = local write "On Time (uS)"(w303) -> ()
              }
            }
            n150 = case shown="True" "PULOFF" {
              tunnel: w283 -> [_ w302]
              frame False {
              }
              frame True {
                n151 = local write "Off Time (uS)"(w302) -> ()
              }
            }
            n152 = case shown="True" "PULNUM" {
              tunnel: w271 -> [_ w301]
              frame False {
              }
              frame True {
                n153 = local write "# of Pulses"(w301) -> ()
              }
            }
          }
          event "KeyPad", "Enter": Value Change {
            n154 = event-data() -> ()  [unwired: 1 in, 5 out]
            n155 = call "Keypad.vi"("KeyPad"="KeyPad") -> ("Keypad Out"=w313:dbl)  [unwired: 14 in]
            "KeyPad Out" <- w313
            n156 = case shown="True" "Enter" {
              tunnel: w313 -> [_ w326]
              tunnel: w312 -> [_ w318]
              frame False {
              }
              frame True {
                n157 = In Range and Coerce(upper limit=4500.0, x=w326, lower limit=34.0) -> (coerced(x)=w316:dbl)  [unwired: 1 out]
                n158 = local write "RF  FREQUENCY MHz"(w316) -> ()
                n159 = local write "Freq (MHz) 3"(w316) -> ()
                n160 = Number To Fractional String(use system decimal point (T)=FALSE, number=w316, precision (6)=i16 3) -> (F-format string=w323:string)  [unwired: 1 in]
                n161 = Concatenate Strings("f" ("element"), w323) -> (w320:string)
                n162 = call "SerialcharWrite.vi"("VISA resource name"=w318, "write buffer"=w320) -> ("ComError"=w317:bool)  [unwired: 8 in]
                n163 = local write "COM Error"(w317) -> ()
              }
            }
          }
          event "Start Frequency", "Stop Frequency", "Step Time (mS)", "Step Size MHz": Value Change {
            # "Set up processor controlled Sweep\nand computer controlled sweep parameters"
            n164 = event-data() -> ()  [unwired: 1 in, 5 out]
            n165 = Subtract(x="Stop Frequency", y="Start Frequency") -> (x-y=w331:dbl)
            n166 = Divide(x=w331, y="Step Size MHz") -> (x/y=→"Number\nof Points":dbl)
            n167 = Number To Fractional String(use system decimal point (T)=FALSE, number="Step Size MHz", precision (6)=i16 3) -> (F-format string=w339:string)  [unwired: 1 in]
            n168 = Number To Fractional String(use system decimal point (T)=FALSE, number="Step Time (mS)", precision (6)=i16 3) -> (F-format string=w335:string)  [unwired: 1 in]
            n169 = Number To Fractional String(use system decimal point (T)=FALSE, number="Start Frequency", precision (6)=i16 3) -> (F-format string=w352:string)  [unwired: 1 in]
            n170 = Number To Fractional String(use system decimal point (T)=FALSE, number="Stop Frequency", precision (6)=i16 3) -> (F-format string=w343:string)  [unwired: 1 in]
            n171 = Concatenate Strings("d0" ("element"), "r0" ("string"), "l" ("element"), w352, "u" ("element"), w343, "s" ("element"), w339, "t" ("element"), w335) -> (w349:string)
            n172 = call "SerialcharWrite.vi"("VISA resource name"=w327, "write buffer"=w349) -> ("ComError"=w353:bool)  [unwired: 8 in]
            n173 = local write "COM Error"(w353) -> ()
          }
          event "On Time (uS)", "Off Time (uS)", "# of Pulses", "Mod Style": Value Change {
            w376 = 500000.0 ("y")
            # "Pulse Modulation"
            n174 = event-data() -> ()  [unwired: 1 in, 5 out]
            n175 = case shown="False" "Mod Style" {
              tunnel: [w380 u8 64] -> w378
              frame False {
                # "(only PDBrf is toggled)"
                # "High Symetry"
                n176 = local read "Attenuator (dB)"() -> (w381:dbl)
                n177 = Multiply(x=w381, y=2.0) -> (x*y=w383:dbl)
                n178 = Add(x=w383, y=63.0) -> (x+y=w385:dbl)
                n179 = To Unsigned Byte Integer(number=w385) -> (unsigned 8bit integer=w380:u8)
              }
              frame True {
                # "PDBrf plus DVGA lines\nare all toggled"
                # "Hi Isolation\nPAM"
              }
            }
            n180 = To Double Precision Float(number="On Time (uS)") -> (double precision float=w362:dbl)
            n181 = To Double Precision Float(number="Off Time (uS)") -> (double precision float=w361:dbl)
            n182 = To Double Precision Float(number="# of Pulses") -> (double precision float=w360:dbl)
            n183 = Add(x=w362, y=w361) -> (x+y=w375:dbl)
            n184 = Number To Decimal String(number="On Time (uS)") -> (decimal integer string=w357:string)  [unwired: 1 in]
            n185 = Number To Decimal String(number="Off Time (uS)") -> (decimal integer string=w358:string)  [unwired: 1 in]
            n186 = Number To Decimal String(number=w378) -> (decimal integer string=w365:string)  [unwired: 1 in]
            n187 = Multiply(x=w375, y=w360) -> (x*y=w371:dbl)
            n188 = Greater?(x=w371, y=w376) -> (0:w373:bool)
            n189 = case shown="True" w373 {
              tunnel: [w387 w389] -> w372
              tunnel: "# of Pulses" -> [w387 _]
              tunnel: w375 -> [_ w390]
              frame False {
              }
              frame True {
                n190 = Divide(x=500000.0 ("y"), y=w390) -> (x/y=w388:dbl)
                n191 = To Unsigned Word Integer(number=w388) -> (unsigned 16bit integer=w389:u16)
              }
            }
            n192 = Number To Decimal String(number=w372) -> (decimal integer string=w359:string)  [unwired: 1 in]
            n193 = Concatenate Strings("P" ("string"), w357, "O" ("string"), w358, "R" ("string"), w359, "M" ("string"), w365) -> (w366:string)
            n194 = call "SerialcharWrite.vi"("VISA resource name"=w354, "write buffer"=w366) -> ("ComError"=w379:bool)  [unwired: 8 in]
            n195 = local write "COM Error"(w379) -> ()
            n196 = In Range and Coerce(upper limit=w376, x=w371, lower limit=0.0) -> (coerced(x)=→"Duration (uS)":dbl)  [unwired: 1 out]
          }
          event "Sweep\nContinuously": Value Change {
            # "Sweep Continuously"
            n197 = event-data() -> ()  [unwired: 1 in, 5 out]
            n198 = Boolean To (0,1)(Boolean="Sweep\nContinuously") -> (0, 1=w400:i16)
            n199 = Number To Decimal String(number=w400) -> (decimal integer string=w396:string)  [unwired: 1 in]
            n200 = Concatenate Strings("d" ("element"), "0" ("element"), "c" ("element"), w396, "g" ("element"), w396) -> (w397:string)
            n201 = call "SerialcharWrite.vi"("VISA resource name"=w401, "write buffer"=w397) -> ("ComError"=w393:bool)  [unwired: 8 in]
            n202 = local write "COM Error"(w393) -> ()
          }
          event "Send\nCal": Value Change {
            n203 = event-data() -> ()  [unwired: 1 in, 5 out]
            n204 = Number To Fractional String(use system decimal point (T)=FALSE, number="VREF", precision (6)=i16 3) -> (F-format string=w409:string)  [unwired: 1 in]
            n205 = Number To Fractional String(use system decimal point (T)=FALSE, number="POFFSET", precision (6)=i16 3) -> (F-format string=w404:string)  [unwired: 1 in]
            n206 = Concatenate Strings("V" ("element"), w409, "Q" ("string"), w404) -> (w412:string)
            n207 = call "SerialcharWrite.vi"("VISA resource name"=w402, "write buffer"=w412) -> ()  [unwired: 8 in, 1 out]
          }
          event "stop": Value Change {
            n208 = event-data() -> ()  [unwired: 1 in, 5 out]
          }
          event "Read Settings\nFrom SynthNV": Value Change {
            n209 = event-data() -> ()  [unwired: 1 in, 5 out]
            n210 = call "SerialCharWriteandRead.vi"("VISA resource name"=w415, "write buffer"="?") -> ("error?"=w416:bool, "read buffer"=→"read buffer":string)  [unwired: 5 in, 2 out]
            n211 = local write "COM Error"(w416) -> ()
          }
          event "Sweep\nOnce": Value Change {
            # "Sweep Once"
            n212 = event-data() -> ()  [unwired: 1 in, 5 out]
            n213 = local read "Stop Frequency"() -> (w419:dbl)
            n214 = Concatenate Strings("d" ("element"), "0" ("element"), "g" ("element"), "1" ("string")) -> (w423:string)
            n215 = call "SerialcharWrite.vi"("VISA resource name"=w426, "write buffer"=w423) -> ("ComError"=w420:bool)  [unwired: 8 in]
            n216 = local write "COM Error"(w420) -> ()
            n217 = local write "RF  FREQUENCY MHz"(w419) -> ()
            n218 = local write "Freq (MHz) 3"(w419) -> ()
          }
          event "Allow changing\nof Power Detector\ncalibration values": Value Change {
            n219 = event-data() -> ()  [unwired: 1 in, 5 out]
            n220 = Select(t=T4."Enabled" ("Disabled"), s="Allow changing\nof Power Detector\ncalibration values", f=T4."Disabled and Grayed Out" ("Disabled")) -> (s? t:f=w428:T4)
            n221 = property on="Send\nCal" class="Bool"("DisabledEnum"=w428) -> ()  [unwired: 2 in, 2 out]
            n222 = property on="VREF" class="DigNum (strict)"("DisabledEnum"=w428) -> ()  [unwired: 2 in, 2 out]
            n223 = property on="POFFSET" class="DigNum (strict)"("DisabledEnum"=w428) -> ()  [unwired: 2 in, 2 out]
          }
          event "Continuous PM": Value Change {
            # "Pulse Continuously"
            n224 = event-data() -> ()  [unwired: 1 in, 5 out]
            n225 = Boolean To (0,1)(Boolean="Continuous PM") -> (0, 1=w436:i16)
            n226 = Select(t=2.0, s="Continuous PM", f=0.0) -> (s? t:f=w440:dbl)
            n227 = property on="Send Pulse Burst" class="Bool"("DisabledEnum"=w440) -> ()  [unwired: 2 in, 2 out]
            n228 = Number To Decimal String(number=w436) -> (decimal integer string=w433:string)  [unwired: 1 in]
            n229 = Concatenate Strings("j" ("element"), w433) -> (w434:string)
            n230 = call "SerialcharWrite.vi"("VISA resource name"=w437, "write buffer"=w434) -> ("ComError"=w432:bool)  [unwired: 8 in]
            n231 = local write "COM Error"(w432) -> ()
          }
          event "Send Pulse Burst": Value Change {
            # "Send Pulse Burst"
            n232 = event-data() -> ()  [unwired: 1 in, 5 out]
            n233 = call "SerialcharWrite.vi"("VISA resource name"=w441, "write buffer"="G") -> ("ComError"=w443:bool)  [unwired: 8 in]
            n234 = local write "COM Error"(w443) -> ()
          }
          event "Continuous AM": Value Change {
            n235 = event-data() -> ()  [unwired: 1 in, 5 out]
            n236 = Select(t=2.0, s="Continuous AM", f=0.0) -> (s? t:f=w452:dbl)
            n237 = property on="Send AM Burst" class="Bool"("DisabledEnum"=w452) -> ()  [unwired: 2 in, 2 out]
            n238 = Boolean To (0,1)(Boolean="Continuous AM") -> (0, 1=w448:i16)
            n239 = Number To Decimal String(number=w448) -> (decimal integer string=w445:string)  [unwired: 1 in]
            n240 = Concatenate Strings("A" ("element"), w445) -> (w446:string)
            n241 = call "SerialcharWrite.vi"("VISA resource name"=w449, "write buffer"=w446) -> ("ComError"=w444:bool)  [unwired: 8 in]
            n242 = local write "COM Error"(w444) -> ()
          }
          event "Send AM Burst": Value Change {
            n243 = event-data() -> ()  [unwired: 1 in, 5 out]
            n244 = call "SerialcharWrite.vi"("VISA resource name"=w456, "write buffer"="B") -> ("ComError"=w454:bool)  [unwired: 8 in]
            n245 = local write "COM Error"(w454) -> ()
          }
          event "LUTsize", "Wave Shape": Value Change {
            # "AM"
            # "Setup Lookup Table for AM"
            n246 = event-data() -> ()  [unwired: 1 in, 5 out]
            n247 = call "AMLUTwaveselect.vi"("Wave Shape"="Wave Shape", "LUTsize"=w457) -> ("Array"=w459:u8[])  [unwired: 1 in]
            n248 = Build Array (concatenate)(u8 9 ("element"), w457, w459) -> (w461:u8[])
            n249 = call "SerialByteWrite.vi"("VISA resource name"=w462, "unsigned byte array"=w461) -> ("error?"=w458:bool)  [unwired: 8 in]
            n250 = local write "COM Error"(w458) -> ()
          }
          event "AM Freq (Hz)", "# of Cycles", "Amplitude (%)", "Offset": Value Change {
            n251 = event-data() -> ()  [unwired: 1 in, 5 out]
            n252 = call "AMFreqminduration.vi"("Offset"="Offset", "Amplitude (%)"="Amplitude (%)", "Reps"="# of Cycles", "AM Freq (Hz)"="AM Freq (Hz)", "LUT size"=w464) -> ("Duration (ms)"=→"Duration (ms)":dbl, "AMout"=w473:string, "Actual Freq"=→"Actual Freq (Hz)":dbl)  [unwired: 4 in]
            n253 = call "SerialcharWrite.vi"("VISA resource name"=w465, "write buffer"=w473) -> ("ComError"=w466:bool)  [unwired: 8 in]
            n254 = local write "COM Error"(w466) -> ()
          }
          event "PllCntrl", "Send", "Freq (MHz)", "Step Size (MHz)": Value Change {
            # "RAW register writes for controlling\nregisters 2,3,5 especially"
            n255 = event-data() -> ()  [unwired: 1 in, 5 out]
            n256 = call "Getsettings.vi"("PllCntrl"="PllCntrl", "Step Size  (MHz)"="Step Size (MHz)", "Freq (MHz)"="Freq (MHz)") -> ("Modulus"=w479:i32, "INT"=w478:i16, "FRAC"=w477:i32, "RF Divider"=w476:i32, "Pfd (MHz)"=→"PFd(MHz)":dbl)  [unwired: 1 in, 2 out]
            "Frac" <- w477
            "Modulus" <- w479
            "INT" <- w478
            "RF Divider" <- w476
            n257 = call "Get Registers.vi"("Out Divider"=w476, "PllCntrl"="PllCntrl", "INT"=w478, "FRAC"=w477, "MOD"=w479) -> ("concatenated string"=w482:string, "Allregout"=→"Allregout":u32[])  [unwired: 13 in]
            n258 = case shown="True" "Send" {
              tunnel: w474 -> [_ w488]
              tunnel: w482 -> [_ w487]
              frame False {
              }
              frame True {
                n259 = call "SerialcharWrite.vi"("VISA resource name"=w488, "write buffer"=w487) -> ("ComError"=w486:bool)  [unwired: 8 in]
                n260 = local write "COM Error"(w486) -> ()
              }
            }
          }
          event "Start Network\nAnalyzer": Value Change {
            n261 = event-data() -> ()  [unwired: 1 in, 5 out]
            n262 = stacked-sequence {
              tunnel: w489 -> [w491 _ _ _ w519 w532 w534]
              frame #0 {
                n263 = local read "Attenuator (dB)"() -> (w492:dbl)
                n264 = Multiply(x=w492, y=2.0) -> (x*y=w498:dbl)
                n265 = Add(x=w498, y=63.0) -> (x+y=w500:dbl)
                n266 = To Unsigned Byte Integer(number=w500) -> (unsigned 8bit integer=w493:u8)
                n267 = Number To Decimal String(number=w493) -> (decimal integer string=w496:string)  [unwired: 1 in]
                n268 = Concatenate Strings("A0j0g0" ("string"), "a" ("element"), w496) -> (w494:string)
                n269 = call "SerialcharWrite.vi"("VISA resource name"=w491, "write buffer"=w494) -> ()  [unwired: 8 in, 1 out]
              }
              frame #1 {
                w501 = T4."Enabled" ("Disabled")
                w502 = TRUE
                w503 = FALSE
                n270 = local write "Sweep\nContinuously"(w503) -> ()
                n271 = local write "Read Power"(w503) -> ()
                n272 = local write "Continuous PM"(w503) -> ()
                n273 = local write "Continuous AM"(w503) -> ()
                n274 = local write "RF HP"(w502) -> ()
                n275 = local write "RF On"(w502) -> ()
                n276 = property on="Send AM Burst" class="Bool"("DisabledEnum"=w501) -> ()  [unwired: 2 in, 2 out]
                n277 = property on="Send Pulse Burst" class="Bool"("DisabledEnum"=w501) -> ()  [unwired: 2 in, 2 out]
              }
              frame #2 {
                n278 = Wait (ms)(milliseconds to wait=u32 100) -> ()  [unwired: 1 out]
              }
              frame #3 {
                w505 = T5 0 items=["no dialog", "OK message", "continue or stop message", "OK message + warnings", "continue/stop + warnings"] ("type of dialog (OK msg:1)")
                n279 = vi-ref "NAfull.vi"() -> (w507:refnum<vi>)
                n280 = property class="VI"(reference=w507) -> ("Name"=w506:string)  [unwired: 1 in, 2 out]
                n281 = Open VI Reference(type specifier VI Refnum (for type only)=refnum<vi> refnum, vi path=w506) -> (vi reference=w513:refnum<vi>, error out=w511:errorcluster)  [unwired: 4 in]
                n282 = call-by-ref "?"(reference=w513, error in=w511) -> (reference out=w510:refnum<vi>, error out=w509:errorcluster)  [unwired: 12 in]
                n283 = Close Reference(reference=w510, error in (no error)=w509) -> (error out=w508:errorcluster)
                n284 = call <vilib>:"Simple Error Handler.vi"("type of dialog (OK msg:1)"=w505, "error in (no error)"=w508) -> ()  [unwired: 3 in, 5 out]
              }
              frame #4 {
                n285 = local read "RF  FREQUENCY MHz"() -> (w518:dbl)
                n286 = Number To Fractional String(use system decimal point (T)=FALSE, number=w518, precision (6)=i16 3) -> (F-format string=w524:string)  [unwired: 1 in]
                n287 = Concatenate Strings("f" ("element"), w524) -> (w521:string)
                n288 = call "SerialcharWrite.vi"("VISA resource name"=w519, "write buffer"=w521) -> ("ComError"=w514:bool)  [unwired: 8 in]
                n289 = Equal?(x=w514, y=TRUE) -> (x = y?=w516:bool)
                n290 = case shown="True" w516 {
                  tunnel: "Serial Port Error" ("message") -> [_ w525]
                  frame False {
                  }
                  frame True {
                    n291 = Two Button Dialog(message=w525) -> ()  [unwired: 2 in, 1 out]
                  }
                }
              }
              frame #5 {
                n292 = call "SerialCharWRtermchar.vi"("VISA resource name"=w532, "write buffer"="a?") -> ("read buffer"=w527:string)  [unwired: 6 in, 2 out]
                n293 = Fract/Exp String To Number(string=w527) -> (number=w528:dbl)  [unwired: 3 in, 1 out]
                n294 = Subtract(x=w528, y=63.0) -> (x-y=w529:dbl)
                n295 = Divide(x=w529, y=2.0) -> (x/y=w526:dbl)
                n296 = local write "Attenuator (dB)"(w526) -> ()
              }
              frame #6 {
                n297 = stacked-sequence {
                  tunnel: w534 -> [w535 w538 w545 w552 w559 w562]
                  frame #0 {
                    # "Open Serial Port"
                    n298 = call-poly "VISA Configure Serial Port"("VISA resource name"=w535, "timeout (10sec)"=u32 1000) -> ()  [unwired: 7 in, 7 out]
                  }
                  frame #1 {
                    # "Get Start Frequency"
                    n299 = call "SerialCharWriteReadnoopen.vi"("VISA resource name"=w538, "write buffer"="l?") -> ("read buffer"=w542:string)  [unwired: 8 in]
                    n300 = Decimal String To Number(string=w542, default (0L)=0.0 ("default (0 I32)")) -> (number=w540:dbl)  [unwired: 1 in, 1 out]
                    n301 = Divide(x=w540, y=1000.0) -> (x/y=w537:dbl)
                    n302 = local write "Start Frequency"(w537) -> ()
                  }
                  frame #2 {
                    # "Get Stop Frequency"
                    n303 = call "SerialCharWriteReadnoopen.vi"("VISA resource name"=w545, "write buffer"="u?") -> ("read buffer"=w549:string)  [unwired: 8 in]
                    n304 = Decimal String To Number(string=w549, default (0L)=0.0 ("default (0 I32)")) -> (number=w547:dbl)  [unwired: 1 in, 1 out]
                    n305 = Divide(x=w547, y=1000.0) -> (x/y=w544:dbl)
                    n306 = local write "Stop Frequency"(w544) -> ()
                  }
                  frame #3 {
                    # "Get Step Size"
                    n307 = call "SerialCharWriteReadnoopen.vi"("VISA resource name"=w552, "write buffer"="s?") -> ("read buffer"=w556:string)  [unwired: 8 in]
                    n308 = Decimal String To Number(string=w556, default (0L)=0.0 ("default (0 I32)")) -> (number=w554:dbl)  [unwired: 1 in, 1 out]
                    n309 = Divide(x=w554, y=1000.0) -> (x/y=w551:dbl)
                    n310 = local write "Step Size MHz"(w551) -> ()
                  }
                  frame #4 {
                    # "Get Step Time"
                    n311 = call "SerialCharWriteReadnoopen.vi"("VISA resource name"=w559, "write buffer"="t?") -> ("read buffer"=w560:string)  [unwired: 8 in]
                    n312 = Fract/Exp String To Number(string=w560) -> (number=w558:dbl)  [unwired: 3 in, 1 out]
                    n313 = local write "Step Time (mS)"(w558) -> ()
                  }
                  frame #5 {
                    w563 = T5 0 items=["no dialog", "OK message", "continue or stop message", "OK message + warnings", "continue/stop + warnings"] ("type of dialog (OK msg:1)")
                    n314 = VISA Close(VISA resource name=w562) -> (error out=w564:errorcluster)  [unwired: 1 in]
                    n315 = call <vilib>:"Simple Error Handler.vi"("type of dialog (OK msg:1)"=w563, "error in (no error)"=w564) -> ()  [unwired: 8 out]
                  }
                }
              }
            }
          }
          event "Re-init\nDefaults": Value Change {
            # "Reinit to defaults"
            n316 = event-data() -> ()  [unwired: 1 in, 5 out]
            n317 = stacked-sequence {
              tunnel: w565 -> [w566 w570 _ w586]
              frame #0 {
                # "Set Reference"
                n318 = call "SerialcharWrite.vi"("VISA resource name"=w566, "write buffer"="x1") -> ()  [unwired: 8 in, 1 out]
              }
              frame #1 {
                n319 = call "SerialcharWrite.vi"("VISA resource name"=w570, "write buffer"="H500580005H400A1043CH3000004B3H218015E42H108008FA1H003E80000") -> ("ComError"=w568:bool)  [unwired: 8 in]
                n320 = local write "COM Error"(w568) -> ()
              }
              frame #2 {
                n321 = local write "Step Size (MHz)"(0.001 ("Step Size (MHz)")) -> ()
                n322 = local write "Freq (MHz)"(1000.0 ("Freq (MHz)")) -> ()
                n323 = local read "PllCntrl"() -> (w571:T3)
                n324 = Bundle By Name(cluster=w571, "PLL PWR"=i8 3, "MUX out"=u16 4, "Phase"=i16 1, "Low Noise"=TRUE, "REF X2"=FALSE, "Mute till LD"=TRUE, "Icp"=15, "Band Sel Div"=16, "REF Divide"=i16 5, "Reference(MHz)"=10.0) -> (w584:T3)
                n325 = local write "PllCntrl"(w584) -> ()
              }
              frame #3 {
                w585 = 1000.0 ("RF  FREQUENCY MHz")
                n326 = local write "RF  FREQUENCY MHz"(w585) -> ()
                n327 = local write "Freq (MHz) 3"(w585) -> ()
                n328 = call "SerialcharWrite.vi"("VISA resource name"=w586, "write buffer"="o1h1f1000.0e") -> ()  [unwired: 8 in, 1 out]
              }
            }
          }
          event "GP Dig Out J8 P3": Value Change {
            n329 = event-data() -> ()  [unwired: 1 in, 5 out]
            n330 = Boolean To (0,1)(Boolean="GP Dig Out J8 P3") -> (0, 1=w591:i16)
            n331 = Number To Decimal String(number=w591) -> (decimal integer string=w590:string)  [unwired: 1 in]
            n332 = Concatenate Strings("#" ("element"), w590) -> (w592:string)
            n333 = call "SerialcharWrite.vi"("VISA resource name"=w594, "write buffer"=w592) -> ("ComError"=w589:bool)  [unwired: 8 in]
            n334 = local write "COM Error"(w589) -> ()
          }
          event "GP Dig Out J8 P5": Value Change {
            n335 = event-data() -> ()  [unwired: 1 in, 5 out]
            n336 = Boolean To (0,1)(Boolean="GP Dig Out J8 P5") -> (0, 1=w598:i16)
            n337 = Number To Decimal String(number=w598) -> (decimal integer string=w597:string)  [unwired: 1 in]
            n338 = Concatenate Strings("$" ("element"), w597) -> (w599:string)
            n339 = call "SerialcharWrite.vi"("VISA resource name"=w595, "write buffer"=w599) -> ("ComError"=w596:bool)  [unwired: 8 in]
            n340 = local write "COM Error"(w596) -> ()
          }
          event "Program\nEEprom": Value Change {
            n341 = event-data() -> ()  [unwired: 1 in, 5 out]
            n342 = call "SerialcharWrite.vi"("VISA resource name"=w602, "write buffer"="e") -> ("ComError"=w603:bool)  [unwired: 8 in]
            n343 = local write "COM Error"(w603) -> ()
          }
          event "Read\nFirmware\nVersion": Value Change {
            n344 = event-data() -> ()  [unwired: 1 in, 5 out]
            n345 = call "SerialCharWRtermchar.vi"("VISA resource name"=w605, "write buffer"="v") -> ("error?"=w606:bool, "read buffer"=→"Version":string)  [unwired: 6 in, 1 out]
            n346 = local write "COM Error"(w606) -> ()
          }
          event "Attenuator (dB)": Value Change {
            # "write to VGA"
            n347 = event-data() -> ()  [unwired: 1 in, 5 out]
            n348 = local read "RF  FREQUENCY MHz"() -> (w615:dbl)
            n349 = local read "caldata"() -> (w614:dbl[][])
            n350 = local read "RF HP"() -> (w612:bool)
            n351 = local read "RF On"() -> (w611:bool)
            n352 = call "getcalpwr.vi"("RF On"=w611, "caldata"=w614, "RF HP"=w612, "attn"="Attenuator (dB)", "freq"=w615) -> ("actual"=→"Power (dBm)":dbl)  [unwired: 5 in]
            n353 = Multiply(x="Attenuator (dB)", y=2.0) -> (x*y=w622:dbl)
            n354 = Add(x=w622, y=63.0) -> (x+y=w624:dbl)
            n355 = To Unsigned Byte Integer(number=w624) -> (unsigned 8bit integer=w610:u8)
            n356 = Number To Decimal String(number=w610) -> (decimal integer string=w620:string)  [unwired: 1 in]
            n357 = Concatenate Strings("a" ("element"), w620) -> (w618:string)
            n358 = call "SerialcharWrite.vi"("VISA resource name"=w616, "write buffer"=w618) -> ("ComError"=w617:bool)  [unwired: 8 in]
            n359 = local write "COM Error"(w617) -> ()
          }
          event "Program\nReference": Value Change {
            n360 = event-data() -> ()  [unwired: 1 in, 5 out]
            n361 = Boolean To (0,1)(Boolean="REF") -> (0, 1=w629:i16)
            n362 = Number To Decimal String(number=w629) -> (decimal integer string=w630:string)  [unwired: 1 in]
            n363 = Concatenate Strings("x" ("write buffer"), w630) -> (w627:string)
            n364 = call "SerialcharWrite.vi"("VISA resource name"=w625, "write buffer"=w627) -> ("ComError"=w626:bool)  [unwired: 8 in]
            n365 = local write "COM Error"(w626) -> ()
          }
          event "RF HP": Value Change {
            n366 = event-data() -> ()  [unwired: 1 in, 5 out]
            n367 = local read "RF  FREQUENCY MHz"() -> (w636:dbl)
            n368 = local read "Attenuator (dB)"() -> (w635:dbl)
            n369 = local read "caldata"() -> (w633:dbl[][])
            n370 = local read "RF On"() -> (w634:bool)
            n371 = Boolean To (0,1)(Boolean="RF HP") -> (0, 1=w641:i16)
            n372 = Number To Decimal String(number=w641) -> (decimal integer string=w640:string)  [unwired: 1 in]
            n373 = call "getcalpwr.vi"("RF On"=w634, "caldata"=w633, "RF HP"="RF HP", "attn"=w635, "freq"=w636) -> ("actual"=w632:dbl)  [unwired: 5 in]
            n374 = Concatenate Strings("h" ("element"), w640) -> (w642:string)
            n375 = call "SerialcharWrite.vi"("VISA resource name"=w638, "write buffer"=w642) -> ("ComError"=w639:bool)  [unwired: 8 in]
            n376 = local write "COM Error"(w639) -> ()
            n377 = local write "Power (dBm)"(w632) -> ()
          }
          event "RF On": Value Change {
            # "Setting Frequency\nMake sure calibration\nHappens even if Powered down"
            n378 = event-data() -> ()  [unwired: 1 in, 5 out]
            n379 = local read "RF  FREQUENCY MHz"() -> (w648:dbl)
            n380 = local read "Attenuator (dB)"() -> (w647:dbl)
            n381 = local read "caldata"() -> (w645:dbl[][])
            n382 = local read "RF HP"() -> (w646:bool)
            n383 = call "getcalpwr.vi"("RF On"="RF On", "caldata"=w645, "RF HP"=w646, "attn"=w647, "freq"=w648) -> ("actual"=w644:dbl)  [unwired: 5 in]
            n384 = stacked-sequence {
              tunnel: w650 -> [w655 _ w660]
              tunnel: "RF On" -> [w654 _ w659]
              tunnel: w648 -> [_ _ w661]
              frame #0 {
                n385 = Boolean To (0,1)(Boolean=w654) -> (0, 1=w653:i16)
                n386 = Number To Decimal String(number=w653) -> (decimal integer string=w652:string)  [unwired: 1 in]
                n387 = Concatenate Strings("o" ("element"), w652) -> (w656:string)
                n388 = call "SerialcharWrite.vi"("VISA resource name"=w655, "write buffer"=w656) -> ("ComError"=w651:bool)  [unwired: 8 in]
                n389 = local write "COM Error"(w651) -> ()
              }
              frame #1 {
                n390 = Wait (ms)(milliseconds to wait=u32 1) -> ()  [unwired: 1 out]
              }
              frame #2 {
                n391 = case shown="True" w659 {
                  tunnel: w661 -> [_ w663]
                  tunnel: w660 -> [_ w662]
                  frame False {
                  }
                  frame True {
                    n392 = Number To Fractional String(use system decimal point (T)=FALSE, number=w663, precision (6)=i16 3) -> (F-format string=w665:string)  [unwired: 1 in]
                    n393 = Concatenate Strings("f" ("element"), w665) -> (w668:string)
                    n394 = call "SerialcharWrite.vi"("VISA resource name"=w662, "write buffer"=w668) -> ("ComError"=w664:bool)  [unwired: 8 in]
                    n395 = local write "COM Error"(w664) -> ()
                  }
                }
              }
            }
            n396 = local write "Power (dBm)"(w644) -> ()
          }
          event "Load", "Boolean": Value Change {
            # "Only send one error."
            # "Scan for Devices"
            # "Load settings from SynthNV"
            n397 = event-data() -> ()  [unwired: 1 in, 5 out]
            n398 = local read "COM Error"() -> (w676:bool)
            n399 = feedback #1() -> (w678:bool)  [unwired: 1 in]
            n400 = Equal?(x=w678, y=FALSE) -> (x = y?=w681:bool)
            n401 = feedback-in #1(w676) -> ()
            n402 = Equal?(x=w676, y=TRUE) -> (x = y?=w680:bool)
            n403 = And(x=w680, y=w681) -> (x .and. y?=w682:bool)
            n404 = Or(x=w682, y="Boolean") -> (x .or. y?=w675:bool)
            n405 = case shown="True" w675 {
              tunnel: [FALSE ("y") w685] -> w673
              frame False {
              }
              frame True {
                n406 = call "getcomport.vi"() -> ("No Devices"=w684:bool, "Port"=w687:string, "Device"=→"Device Under Control":string)  [unwired: 9 in]
                n407 = local write "Serial Port Select"(w687) -> ()
                n408 = Not(x=w684) -> (.not. x?=w685:bool)
              }
            }
            n409 = Or(x="Load", y=w673) -> (x .or. y?=w671:bool)
            n410 = case shown="True" w671 {
              tunnel: w670 -> [_ w689]
              frame False {
              }
              frame True {
                n411 = local read "Serial Port Select"() -> (w688:refnum<visa-resource-name>)
                n412 = stacked-sequence {
                  tunnel: w688 -> [w691 w698 w709 w713 w718 w725 w732 w740 w743 w749 w753 w758 w763 w767 w773 w795 w827]
                  tunnel: w689 -> [_ _ _ _ _ _ _ _ _ _ _ _ _ _ _ w794 _]
                  frame #0 {
                    # "Open Serial Port"
                    n413 = call-poly "VISA Configure Serial Port"("VISA resource name"=w691, "timeout (10sec)"=u32 1000) -> ()  [unwired: 7 in, 7 out]
                  }
                  frame #1 {
                    # "Get Frequency"
                    n414 = call "SerialCharWriteReadnoopen.vi"("VISA resource name"=w698, "write buffer"="f?") -> ("read buffer"=w696:string)  [unwired: 8 in]
                    n415 = Decimal String To Number(string=w696, default (0L)=0.0 ("default (0 I32)")) -> (number=w694:dbl)  [unwired: 1 in, 1 out]
                    n416 = Divide(x=w694, y=1000.0) -> (x/y=w692:dbl)
                    n417 = local write "RF  FREQUENCY MHz"(w692) -> ()
                    n418 = local write "Freq (MHz) 3"(w692) -> ()
                  }
                  frame #2 {
                    # "Get Power Slider Setting"
                    n419 = local read "RF  FREQUENCY MHz"() -> (w702:dbl)
                    n420 = local read "caldata"() -> (w703:dbl[][])
                    n421 = local read "RF HP"() -> (w701:bool)
                    n422 = local read "RF On"() -> (w700:bool)
                    n423 = call "SerialCharWriteReadnoopen.vi"("VISA resource name"=w709, "write buffer"="a?") -> ("read buffer"=w710:string)  [unwired: 8 in]
                    n424 = Fract/Exp String To Number(string=w710) -> (number=w705:dbl)  [unwired: 3 in, 1 out]
                    n425 = Subtract(x=w705, y=63.0) -> (x-y=w706:dbl)
                    n426 = Divide(x=w706, y=2.0) -> (x/y=w699:dbl)
                    n427 = call "getcalpwr.vi"("RF On"=w700, "caldata"=w703, "RF HP"=w701, "attn"=w699, "freq"=w702) -> ("actual"=w704:dbl)  [unwired: 5 in]
                    n428 = local write "Power (dBm)"(w704) -> ()
                    n429 = local write "Attenuator (dB)"(w699) -> ()
                  }
                  frame #3 {
                    # "Get Int/Ext Reference"
                    n430 = call "SerialCharWriteReadnoopen.vi"("VISA resource name"=w713, "write buffer"="x?") -> ("read buffer"=w715:string)  [unwired: 8 in]
                    n431 = Decimal String To Number(string=w715) -> (number=w714:i32)  [unwired: 2 in, 1 out]
                    n432 = Not Equal To 0?(x=w714) -> (x != 0?=w712:bool)
                    n433 = local write "REF"(w712) -> ()
                  }
                  frame #4 {
                    # "Get Start Frequency"
                    n434 = call "SerialCharWriteReadnoopen.vi"("VISA resource name"=w718, "write buffer"="l?") -> ("read buffer"=w722:string)  [unwired: 8 in]
                    n435 = Decimal String To Number(string=w722, default (0L)=0.0 ("default (0 I32)")) -> (number=w720:dbl)  [unwired: 1 in, 1 out]
                    n436 = Divide(x=w720, y=1000.0) -> (x/y=w717:dbl)
                    n437 = local write "Start Frequency"(w717) -> ()
                  }
                  frame #5 {
                    # "Get Stop Frequency"
                    n438 = call "SerialCharWriteReadnoopen.vi"("VISA resource name"=w725, "write buffer"="u?") -> ("read buffer"=w729:string)  [unwired: 8 in]
                    n439 = Decimal String To Number(string=w729, default (0L)=0.0 ("default (0 I32)")) -> (number=w727:dbl)  [unwired: 1 in, 1 out]
                    n440 = Divide(x=w727, y=1000.0) -> (x/y=w724:dbl)
                    n441 = local write "Stop Frequency"(w724) -> ()
                  }
                  frame #6 {
                    # "Get Step Size"
                    n442 = call "SerialCharWriteReadnoopen.vi"("VISA resource name"=w732, "write buffer"="s?") -> ("read buffer"=w736:string)  [unwired: 8 in]
                    n443 = Decimal String To Number(string=w736, default (0L)=0.0 ("default (0 I32)")) -> (number=w734:dbl)  [unwired: 1 in, 1 out]
                    n444 = Divide(x=w734, y=1000.0) -> (x/y=w731:dbl)
                    n445 = local write "Step Size MHz"(w731) -> ()
                  }
                  frame #7 {
                    # "Get Step Time"
                    n446 = call "SerialCharWriteReadnoopen.vi"("VISA resource name"=w740, "write buffer"="t?") -> ("read buffer"=w739:string)  [unwired: 8 in]
                    n447 = Fract/Exp String To Number(string=w739) -> (number=w738:dbl)  [unwired: 3 in, 1 out]
                    n448 = local write "Step Time (mS)"(w738) -> ()
                  }
                  frame #8 {
                    n449 = call "SerialCharWriteReadnoopen.vi"("VISA resource name"=w743, "write buffer"="c?") -> ("read buffer"=w745:string)  [unwired: 8 in]
                    n450 = Decimal String To Number(string=w745) -> (number=w744:i32)  [unwired: 2 in, 1 out]
                    n451 = Not Equal To 0?(x=w744) -> (x != 0?=w742:bool)
                    n452 = local write "Sweep\nContinuously"(w742) -> ()
                  }
                  frame #9 {
                    # "Get RF on or off"
                    n453 = call "SerialCharWriteReadnoopen.vi"("VISA resource name"=w749, "write buffer"="o?") -> ("read buffer"=w750:string)  [unwired: 8 in]
                    n454 = Decimal String To Number(string=w750) -> (number=w747:i32)  [unwired: 2 in, 1 out]
                    n455 = Not Equal To 0?(x=w747) -> (x != 0?=w748:bool)
                    n456 = local write "RF On"(w748) -> ()
                  }
                  frame #10 {
                    # "Get RF high power\n or low power"
                    n457 = call "SerialCharWriteReadnoopen.vi"("VISA resource name"=w753, "write buffer"="h?") -> ("read buffer"=w755:string)  [unwired: 8 in]
                    n458 = Decimal String To Number(string=w755) -> (number=w754:i32)  [unwired: 2 in, 1 out]
                    n459 = Not Equal To 0?(x=w754) -> (x != 0?=w752:bool)
                    n460 = local write "RF HP"(w752) -> ()
                  }
                  frame #11 {
                    # "Get Pulse continuously\n (automatically)?"
                    n461 = call "SerialCharWriteReadnoopen.vi"("VISA resource name"=w758, "write buffer"="j?") -> ("read buffer"=w760:string)  [unwired: 8 in]
                    n462 = Decimal String To Number(string=w760) -> (number=w759:i32)  [unwired: 2 in, 1 out]
                    n463 = Not Equal To 0?(x=w759) -> (x != 0?=w757:bool)
                    n464 = local write "Continuous PM"(w757) -> ()
                  }
                  frame #12 {
                    n465 = call "SerialCharWriteReadnoopen.vi"("VISA resource name"=w763, "write buffer"="V?") -> ("read buffer"=w764:string)  [unwired: 8 in]
                    n466 = Fract/Exp String To Number(string=w764) -> (number=w762:dbl)  [unwired: 3 in, 1 out]
                    n467 = local write "VREF"(w762) -> ()
                  }
                  frame #13 {
                    n468 = call "SerialCharWriteReadnoopen.vi"("VISA resource name"=w767, "write buffer"="Q?") -> ("read buffer"=w768:string)  [unwired: 8 in]
                    n469 = Fract/Exp String To Number(string=w768) -> (number=w766:dbl)  [unwired: 3 in, 1 out]
                    n470 = local write "POFFSET"(w766) -> ()
                  }
                  frame #14 {
                    # "Get pulse settings"
                    n471 = stacked-sequence {
                      tunnel: w773 -> [w776 w781 w786]
                      tunnel: [w774 _ _] -> w772
                      tunnel: [_ w780 _] -> w771
                      tunnel: [_ _ w785] -> w770
                      frame #0 {
                        n472 = call "SerialCharWriteReadnoopen.vi"("VISA resource name"=w776, "write buffer"="P?") -> ("read buffer"=w777:string)  [unwired: 8 in]
                        n473 = Decimal String To Number(string=w777, default (0L)=u16 0 ("default (0 I32)")) -> (number=w774:u16)  [unwired: 1 in, 1 out]
                      }
                      frame #1 {
                        n474 = call "SerialCharWriteReadnoopen.vi"("VISA resource name"=w781, "write buffer"="O?") -> ("read buffer"=w782:string)  [unwired: 8 in]
                        n475 = Decimal String To Number(string=w782, default (0L)=u16 0 ("default (0 I32)")) -> (number=w780:u16)  [unwired: 1 in, 1 out]
                      }
                      frame #2 {
                        n476 = call "SerialCharWriteReadnoopen.vi"("VISA resource name"=w786, "write buffer"="R?") -> ("read buffer"=w787:string)  [unwired: 8 in]
                        n477 = Decimal String To Number(string=w787, default (0L)=u16 0 ("default (0 I32)")) -> (number=w785:u16)  [unwired: 1 in, 1 out]
                      }
                    }
                    n478 = local write "Off Time (uS)"(w771) -> ()
                    n479 = local write "On Time (uS)"(w772) -> ()
                    n480 = local write "# of Pulses"(w770) -> ()
                  }
                  frame #15 {
                    # "Get AM settings"
                    n481 = stacked-sequence {
                      tunnel: w795 -> [w803 w808 w813 w817 w821]
                      tunnel: [_ w807 _ _ _] -> w792
                      tunnel: [_ _ w812 _ _] -> w791
                      tunnel: [_ _ _ w816 _] -> w790
                      tunnel: w794 -> [w801 _ _ _ _]
                      tunnel: [w796 _ _ _ _] -> w793
                      tunnel: [_ _ _ _ w822] -> w789
                      frame #0 {
                        n482 = call "SerialCharWriteReadnoopen.vi"("VISA resource name"=w803, "write buffer"="F?") -> ("read buffer"=w804:string)  [unwired: 8 in]
                        n483 = Decimal String To Number(string=w804, default (0L)=u16 0 ("default (0 I32)")) -> (number=w800:u16)  [unwired: 1 in, 1 out]
                        n484 = Multiply(x=w800, y=w801) -> (x*y=w799:u16)
                        n485 = Reciprocal(x=w799) -> (1/x=w798:dbl)
                        n486 = Multiply(x=w798, y=1000000.0) -> (x*y=w796:dbl)
                      }
                      frame #1 {
                        n487 = call "SerialCharWriteReadnoopen.vi"("VISA resource name"=w808, "write buffer"="q?") -> ("read buffer"=w809:string)  [unwired: 8 in]
                        n488 = Decimal String To Number(string=w809, default (0L)=u16 0 ("default (0 I32)")) -> (number=w807:u16)  [unwired: 1 in, 1 out]
                      }
                      frame #2 {
                        n489 = call "SerialCharWriteReadnoopen.vi"("VISA resource name"=w813, "write buffer"="%?") -> ("read buffer"=w814:string)  [unwired: 8 in]
                        n490 = Decimal String To Number(string=w814, default (0L)=u16 0 ("default (0 I32)")) -> (number=w812:u16)  [unwired: 1 in, 1 out]
                      }
                      frame #3 {
                        n491 = call "SerialCharWriteReadnoopen.vi"("VISA resource name"=w817, "write buffer"="@?") -> ("read buffer"=w819:string)  [unwired: 8 in]
                        n492 = Decimal String To Number(string=w819, default (0L)=u16 0 ("default (0 I32)")) -> (number=w816:u16)  [unwired: 1 in, 1 out]
                      }
                      frame #4 {
                        # "Cont AM"
                        n493 = call "SerialCharWriteReadnoopen.vi"("VISA resource name"=w821, "write buffer"="A?") -> ("read buffer"=w824:string)  [unwired: 8 in]
                        n494 = Decimal String To Number(string=w824) -> (number=w825:i32)  [unwired: 2 in, 1 out]
                        n495 = Not Equal To 0?(x=w825) -> (x != 0?=w822:bool)
                      }
                    }
                    n496 = local write "AM Freq (Hz)"(w793) -> ()
                    n497 = local write "Amplitude (%)"(w791) -> ()
                    n498 = local write "# of Cycles"(w792) -> ()
                    n499 = local write "Continuous AM"(w789) -> ()
                    n500 = local write "Offset"(w790) -> ()
                  }
                  frame #16 {
                    w831 = T5 0 items=["no dialog", "OK message", "continue or stop message", "OK message + warnings", "continue/stop + warnings"] ("type of dialog (OK msg:1)")
                    # "Close session to port."
                    n501 = VISA Close(VISA resource name=w827) -> (error out=w832:errorcluster)  [unwired: 1 in]
                    n502 = call <vilib>:"Simple Error Handler.vi"("type of dialog (OK msg:1)"=w831, "error in (no error)"=w832) -> ("error?"=w826:bool)  [unwired: 7 out]
                    n503 = Equal?(x=w826, y=TRUE) -> (x = y?=w829:bool)
                    n504 = case shown="True" w829 {
                      tunnel: "Serial Port Error" ("message") -> [_ w833]
                      frame False {
                      }
                      frame True {
                        n505 = Two Button Dialog(message=w833) -> ()  [unwired: 2 in, 1 out]
                      }
                    }
                  }
                }
              }
            }
          }
          event Panel Close? {
            w835 = TRUE ("Discard?")
            n506 = event-data() -> ("VIRef"=w836:refnum<vi>)  [unwired: 1 in]
            n507 = Close Reference(reference=w836) -> ()  [unwired: 1 in, 1 out]
            n508 = event-data("Discard?"=w835) -> ()  [unwired: 1 in, 1 out]
          }
          event Timeout {
            n509 = event-data() -> ()  [unwired: 1 in, 2 out]
            n510 = stacked-sequence {
              tunnel: w841 -> [w843 w853 w870 w876 w882]
              tunnel: w840 -> [_ _ _ _ w881]
              tunnel: w839 -> [w842 _ _ _ _]
              tunnel: w838 -> [_ _ w869 _ _]
              tunnel: w837 -> [_ _ _ w875 _]
              frame #0 {
                # "RF Detector vs Time Routine"
                n511 = case shown="True" w842 {
                  tunnel: w843 -> [_ w851]
                  frame False {
                    n512 = Wait (ms)(milliseconds to wait=u32 10) -> ()  [unwired: 1 out]
                  }
                  frame True {
                    # "Measure Pwr"
                    n513 = call "SerialCharWRtermchar.vi"("VISA resource name"=w851, "write buffer"="w") -> ("error?"=w845:bool, "read buffer"=w850:string)  [unwired: 6 in, 1 out]
                    n514 = local write "COM Error"(w845) -> ()
                    n515 = Fract/Exp String To Number(string=w850) -> (number=w848:dbl)  [unwired: 3 in, 1 out]
                    "RF Detector Pwr dBm" <- w848
                    "Waveform Chart" <- w848
                    n516 = Greater?(x=w848, y=10.0) -> (0:→"PWR Level":bool)
                  }
                }
              }
              frame #1 {
                # "Poll every second for Phase Lock"
                n517 = case shown="True" "Poll for\nPhase Lock" {
                  tunnel: w853 -> [_ w860]
                  frame False {
                    n518 = property on="Lock" class="Bool (strict)"("Visible"=FALSE) -> ()  [unwired: 2 in, 2 out]
                  }
                  frame True {
                    n519 = Get Date/Time In Seconds() -> (seconds since 1Jan1904=w856:timestamp)
                    n520 = To Double Precision Float(number=w856) -> (double precision float=w858:dbl)
                    n521 = feedback #2() -> (w857:dbl)  [unwired: 1 in]
                    n522 = Round Toward -Infinity(1:w858) -> (0:w859:dbl)
                    n523 = feedback-in #2(w859) -> ()
                    n524 = Not Equal?(x=w859, y=w857) -> (x != y?=w855:bool)
                    n525 = case shown="True" w855 {
                      tunnel: w860 -> [_ w862]
                      frame False {
                      }
                      frame True {
                        n526 = call "SerialCharWRtermchar.vi"("VISA resource name"=w862, "write buffer"="p") -> ("error?"=w863:bool, "read buffer"=w864:string)  [unwired: 6 in, 1 out]
                        n527 = Fract/Exp String To Number(string=w864) -> (number=w868:dbl)  [unwired: 3 in, 1 out]
                        n528 = local write "COM Error"(w863) -> ()
                        n529 = Not Equal?(x=0.0, y=w868) -> (x != y?=→"Lock":bool)
                        n530 = property on="Lock" class="Bool (strict)"("Visible"=TRUE) -> ()  [unwired: 2 in, 2 out]
                      }
                    }
                  }
                }
              }
              frame #2 {
                n531 = case shown="True" w869 {
                  tunnel: w870 -> [_ w871]
                  frame False {
                  }
                  frame True {
                    n532 = call "SerialCharWRtermchar.vi"("VISA resource name"=w871, "write buffer"="C1") -> ("error?"=w872:bool, "read buffer"=→"A/D1":string)  [unwired: 6 in, 1 out]
                    n533 = local write "COM Error"(w872) -> ()
                  }
                }
              }
              frame #3 {
                n534 = case shown="True" w875 {
                  tunnel: w876 -> [_ w877]
                  frame False {
                  }
                  frame True {
                    n535 = call "SerialCharWRtermchar.vi"("VISA resource name"=w877, "write buffer"="C2") -> ("error?"=w880:bool, "read buffer"=→"A/D2":string)  [unwired: 6 in, 1 out]
                    n536 = local write "COM Error"(w880) -> ()
                  }
                }
              }
              frame #4 {
                n537 = case shown="True" w881 {
                  tunnel: w882 -> [_ w884]
                  frame False {
                  }
                  frame True {
                    w883 = T6 128 items=["Flush Receive Buffer"=16, "Write Transmit Buffer to Device"=32, "Flush Receive Buffer (No I/O)"=64, "Flush Transmit Buffer"=128] ("Mask")
                    w886 = T6 64 items=["Flush Receive Buffer"=16, "Write Transmit Buffer to Device"=32, "Flush Receive Buffer (No I/O)"=64, "Flush Transmit Buffer"=128] ("Mask")
                    n538 = VISA Flush I/O Buffer(VISA resource name=w884, mask (16)=w886) -> (error out=w885:errorcluster)  [unwired: 1 in, 1 out]
                    n539 = VISA Flush I/O Buffer(VISA resource name=w884, mask (16)=w883, error in (no error)=w885) -> ()  [unwired: 2 out]
                  }
                }
              }
            }
          }
        }
      }
    }
    frame #3 {
      n540 = case shown="False" w887 {
        frame False {
          n541 = Open VI Reference(vi path=path "SynthNV_2_5c.vi") -> (vi reference=w889:refnum<vi>)  [unwired: 5 in, 1 out]
          n542 = invoke class="VI" method="FP.Close"(reference=w889) -> ()  [unwired: 2 in, 3 out]
        }
        frame True {
        }
      }
    }
  }
